vi "Kpro Globals.vi"() -> ()   [LabVIEW 2016]
panel:
  in  "Pressure Offset":dbl
  out "Profile ID":string="WP-01"
  in  "KPRO Box Number":dbl=800.0
  in  "increment_amount":dbl=-0.1 format="%.2f"
  in  "height_of_box":dbl format="%.2f"
  in  "Reservoir Pressure":dbl=33.8 format="%.2f"
  out "Current Depth":sgl format="%.2f"
  out "Distance":dbl format="%.2f"
  in  "Atmospheric Pressure":dbl format="%.2f"
  in  "Depth to Water Table":dbl format="%.2f"
  in  "Ion Offset":dbl format="%.2f"
  in  "Ion Slope":dbl=44.04 format="%.2f"
  in  "Pressure \nSlope":dbl=24.27199935913086 format="%.2f"
  in  "Flow Slope":dbl=37.99800109863281 format="%.2f"
  in  "String Pot \nSlope":dbl=1.7339999675750732 format="%.2f"
  in  "KPRO Com Port":i32=1
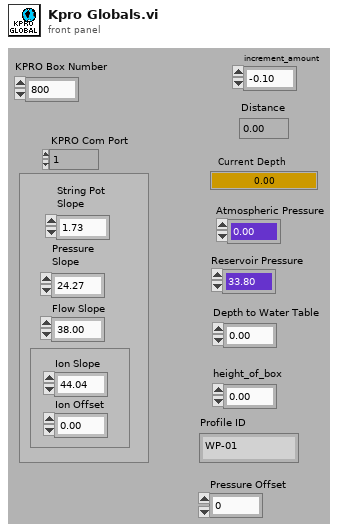
[diagram p1: front panel]
diagram:
